vi "Run Test.vi"(8 "error in (no error)":errorcluster, 11 "CCT Test in":refnum<class "CTT Battery Test.lvclass">) -> (0 "error out":errorcluster, 1 "Fail Codes":string[](array[string]), 2 "Tests Passed":bool[](array[boolean]), 3 "CCT Test out":refnum<class "CTT Battery Test.lvclass">)   [LabVIEW 2015, in "CTT Battery Test.lvclass"]
uses:
  CTT Battery Test.lvclass
  Test Class/Test Class.lvclass
  Classes/Application/Class/Application.lvclass
  CT Common Tests/CT Common Tests.lvclass
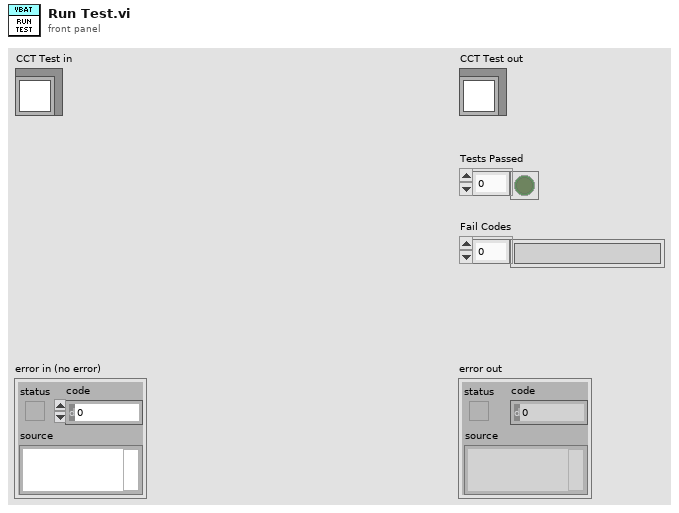
[diagram p1: front panel]
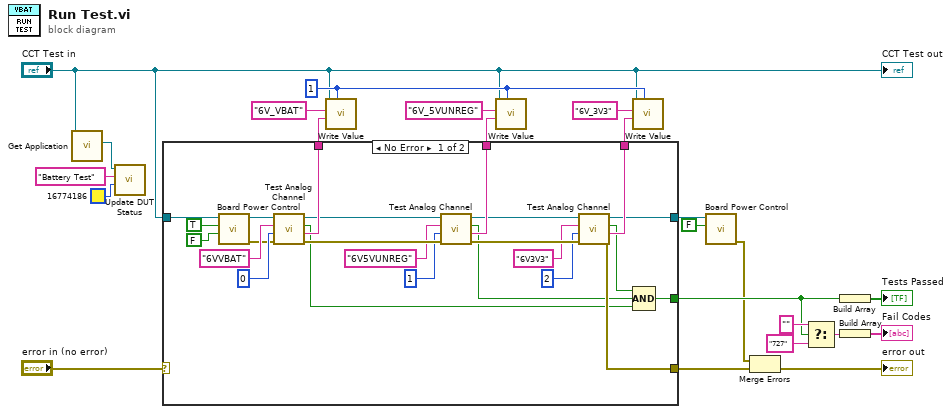
[diagram p0: block diagram]
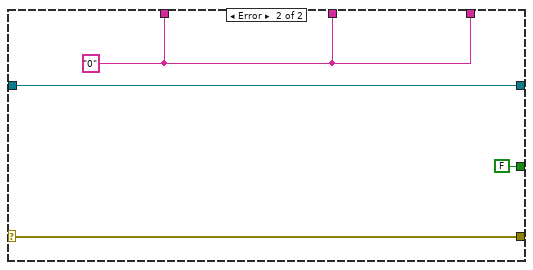
[diagram p2: hidden frame]
diagram:
  w14 = 1 ("DUT")
  n1 = call "Get Application.vi"("Test Class in"="CCT Test in") -> ("Application.lvlib:Application.lvclass"=w10:refnum<class "Application.lvclass">)  [unwired: 9 in, 1 out]
  n2 = call "Update DUT Status.vi"("BG Color"=u32 16774186, "Message ('')"="Battery Test", "Application in"=w10) -> ()  [unwired: 7 in, 2 out]
  n3 = case shown="No Error" "error in (no error)" {
    selector: "error in (no error)" -> [_ w51]
    tunnel: [w47 w51] -> w7
    tunnel: [w39 w49] -> w21
    tunnel: [w34 w49] -> w20
    tunnel: [w29 w49] -> w19
    tunnel: [w44 FALSE] -> w16
    tunnel: "CCT Test in" -> [w26 w48]
    tunnel: [w27 w48] -> w8
    frame No Error {
      n4 = call "Board Power Control.vi"("VBUS"=FALSE, "Power-On"=TRUE, "CT Common Tests"=w26) -> ("error out"=w24:errorcluster, "CT Common Tests"=w25:refnum<class "CTT Battery Test.lvclass">)  [unwired: 7 in]
      n5 = call "Test Analog Channel.vi"("error in (no error)"=w24, "Channel (0)"=u32 0, "Test Label"="6VVBAT", "CT Common Tests in"=w25) -> ("error out"=w45:errorcluster, "Result"=w39:string, "Passed"=w38:bool, "CT Common Tests out"=w37:refnum<class "CTT Battery Test.lvclass">)  [unwired: 4 in]
      n6 = call "Test Analog Channel.vi"("error in (no error)"=w45, "Channel (0)"=u32 1, "Test Label"="6V5VUNREG", "CT Common Tests in"=w37) -> ("error out"=w46:errorcluster, "Result"=w34:string, "Passed"=w33:bool, "CT Common Tests out"=w32:refnum<class "CTT Battery Test.lvclass">)  [unwired: 4 in]
      n7 = call "Test Analog Channel.vi"("error in (no error)"=w46, "Channel (0)"=u32 2, "Test Label"="6V3V3", "CT Common Tests in"=w32) -> ("error out"=w47:errorcluster, "Result"=w29:string, "Passed"=w28:bool, "CT Common Tests out"=w27:refnum<class "CTT Battery Test.lvclass">)  [unwired: 4 in]
      n8 = Compound Arithmetic op=AND(w28, w33, w38) -> (w44:bool)
    }
    frame Error {
      w49 = "0" ("Test Label")
    }
  }
  n9 = call "Write Value.vi"("Position"=w14, "Value"=w21, "Label"="6V_VBAT" ("Test Label"), "Test Class in"="CCT Test in") -> ()  [unwired: 7 in, 1 out]
  n10 = call "Write Value.vi"("Position"=w14, "Value"=w20, "Label"="6V_5VUNREG" ("Test Label"), "Test Class in"="CCT Test in") -> ()  [unwired: 7 in, 1 out]
  n11 = call "Write Value.vi"("Position"=w14, "Value"=w19, "Label"="6V_3V3" ("Test Label"), "Test Class in"="CCT Test in") -> ()  [unwired: 7 in, 1 out]
  n12 = call "Board Power Control.vi"("Power-On"=FALSE, "CT Common Tests"=w8) -> ("error out"=w5:errorcluster)  [unwired: 8 in, 1 out]
  n13 = Merge Errors(w5, w7) -> (→"error out":errorcluster)
  n14 = Select(t="", s=w16, f="727") -> (s? t:f=w15:string)
  n15 = Build Array(w16) -> (→"Tests Passed":bool[])
  n16 = Build Array(w15) -> (→"Fail Codes":string[])
  "CCT Test out" <- "CCT Test in"
